vi "Link Channels.vi"(7 "gRPC ID in":T4, 8 "error in (no error)":errorcluster, 10 "Channels":T1[](array[typedef]), 11 "CIFCorePlugin in":refnum<class "CIFCorePlugin.lvclass">) -> (0 "error out":errorcluster, 3 "CIFCorePlugin out":refnum<class "CIFCorePlugin.lvclass">)   [LabVIEW 2021, in "Template Test Helpers.lvlib"]
uses:
  Template Test Helpers.lvlib
  <vilib>/CIF Foundation/CIF Core/CIFCore/Grpc/CIFCoreWrapper/CIFCoreWrapper.lvlib
  <vilib>/CIF Foundation/CIF Channels Core/ChannelCommon/ChannelCommon.lvlib
  <vilib>/CIF Foundation/CIF Channels Core/ChannelCommon/typedef/New FIFO Instance Configuration.ctl
  <vilib>/CIF Foundation/CIF Channels Core/CIFChannels/CIFChannels.lvclass
  <vilib>/CIF Foundation/CIF Core/CIFCore/Grpc/CIFCoreChannel_client/RPC Messages/cif_channelcore_ConnectSubscriber.ctl
  <vilib>/CIF Foundation/CIF Core/CIFCore/Grpc/CIFCoreChannel_client/CIFCoreChannel_client.lvlib
  <vilib>/CIF Foundation/CIF Core/CIFCore/Common/Typedef/FIFO Publisher.ctl
  <vilib>/CIF Foundation/CIF Core/CIFCore/Common/CIFCoreCommon.lvlib
  <vilib>/CIF Foundation/CIF Core/CIFCore/Class/CIFCorePlugin.lvclass
  <vilib>/gRPC/LabVIEW gRPC Library/Shared/grpcId.ctl
  <vilib>/gRPC/LabVIEW gRPC Library/grpc-lvsupport-release.lvlib
  <vilib>/CIF Foundation/CIF Core/CIFCore/Grpc/CIFCoreChannel_client/RPC Messages/cif_channelcore_PATTERN.ctl
  <vilib>/CIF Foundation/CIF Core/CIFCore/Grpc/CIFCoreChannel_client/RPC Messages/cif_channelcore_Direction.ctl
  <vilib>/CIF Foundation/CIF Core/CIFCore/Grpc/CIFCoreChannel_client/RPC Messages/cif_channelcore_Channel.ctl
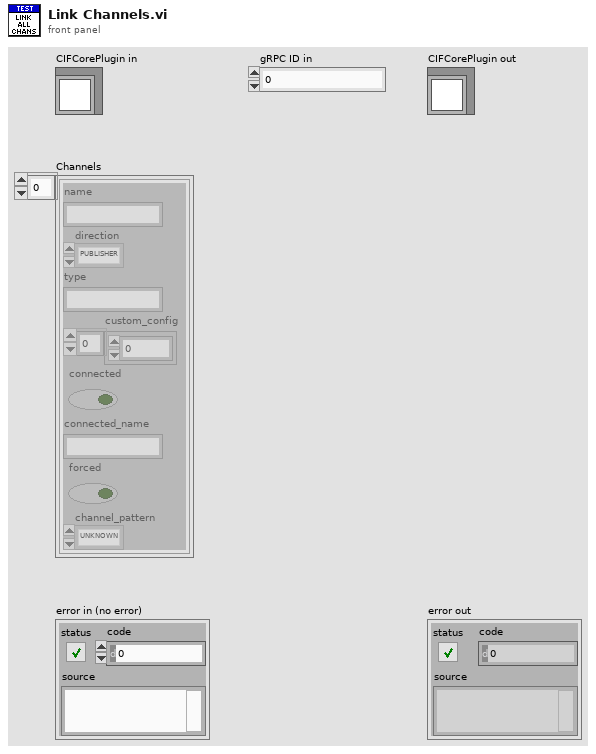
[diagram p1: front panel]
types:
  T1 = typedef "CIFCoreChannel_client.lvlib/cif_channelcore_Channel.ctl" = cluster{"name":string, "direction":T2, "type":string, "custom_config":u8[], "connected":bool, "connected_name":string, "forced":bool, "channel_pattern":T3}
  T2 = typedef "CIFCoreChannel_client.lvlib/cif_channelcore_Direction.ctl" = enum32{"PUBLISHER", "SUBSCRIBER"}
  T3 = typedef "CIFCoreChannel_client.lvlib/cif_channelcore_PATTERN.ctl" = enum32{"UNKNOWN", "TAG", "FIFO", "MULTIFIFO", "BACKPRESSUREFIFO"}
  T4 = typedef "grpc-lvsupport-release.lvlib/grpcId.ctl" = u64
  T5 = typedef "CIFCoreCommon.lvlib/FIFO Publisher.ctl" = cluster{"Publisher Name":string, "New FIFO Instance Config":T6}
  T6 = typedef "ChannelCommon.lvlib/New FIFO Instance Configuration.ctl" = cluster{"Backpressure":bool, "Bytes/Message Override":u32, "Messages/FIFO Override":u32, "Custom Data":u8[]}
  T7 = typedef "CIFCoreChannel_client.lvlib/cif_channelcore_ConnectSubscriber.ctl" = cluster{"subscriber_name":string, "publisher_name":string, "custom_connect":u8[]}
  T8 = typedef "CIFChannels.lvclass/Direction.ctl" = enum16{"Publisher", "Subscriber"}
  T9 = typedef "ChannelCommon.lvlib/FIFO Config.ctl" = cluster{"Max Bytes/Msg":u64, "Max Msg/FIFO":u64, "Flags":u64, "Custom Data":u8[]}
  T10 = typedef "ChannelCommon.lvlib/FIFO Flags.ctl" = cluster{"Backpressure":bool}
  T11 = typedef "ChannelCommon.lvlib/New FIFO Instance Response.ctl" = cluster{"Publisher":string, "Custom Data":u8[]}
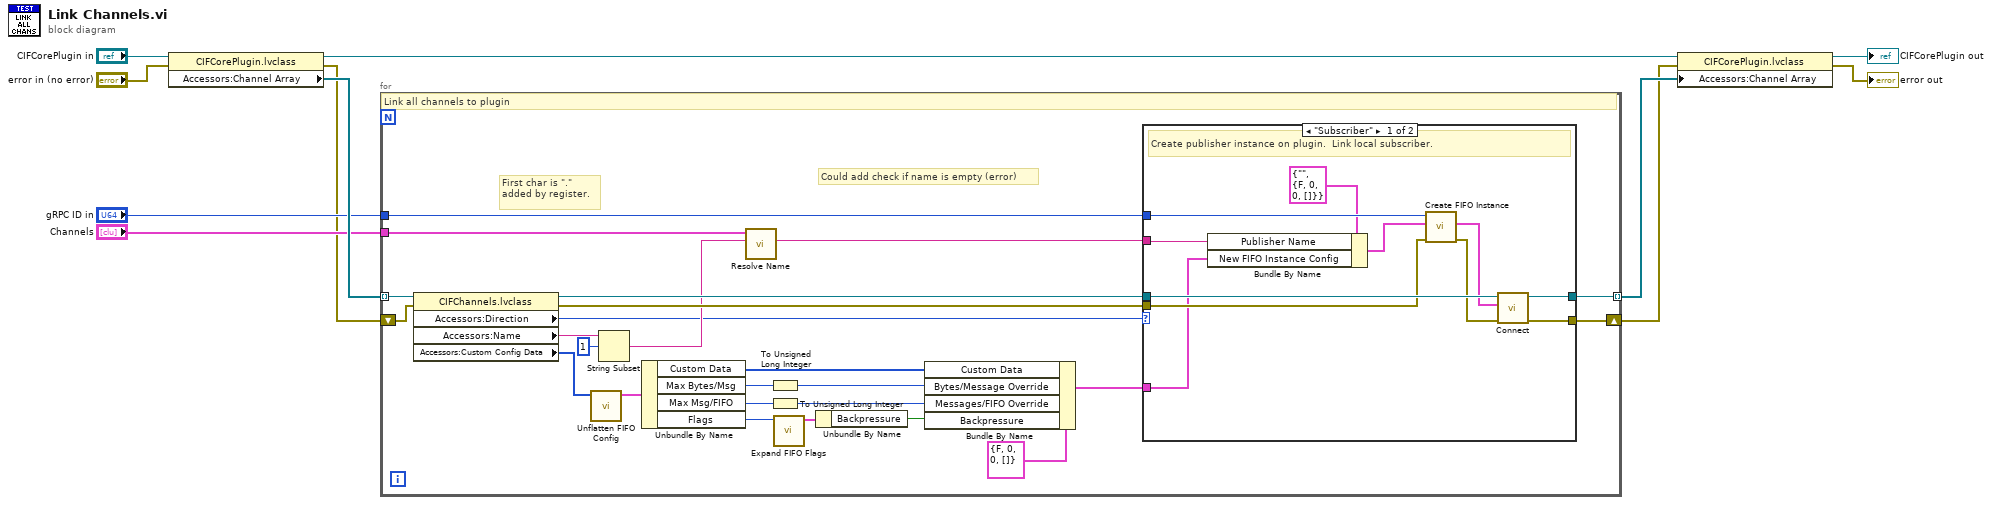
[diagram p0: block diagram]
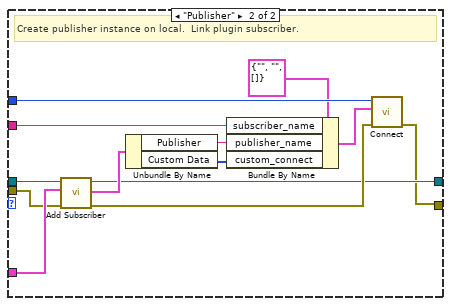
[diagram p2: hidden frame]
diagram:
  n1 = property class="CIFCorePlugin.lvclass"(reference="CIFCorePlugin in", error in="error in (no error)") -> (reference out=w5:refnum<class "CIFCorePlugin.lvclass">, error out=w6:errorcluster, "Accessors:Channel Array"=w10:refnum<class "CIFChannels.lvclass">[])
  n2 = for {
    tunnel: w10 -> [w35] mode=indexing
    tunnel: "Channels" -> [w32]
    tunnel: "gRPC ID in" -> [w31]
    tunnel: [w28] -> w4 mode=indexing
    shift-right: [w27] -> w2
    shift-left: w6 -> [w30]
    w14 = T6 {"Backpressure"=FALSE, "Bytes/Message Override"=0, "Messages/FIFO Override"=0, "Custom Data"=[]} ("New FIFO Instance Config")
    # "Could add check if name is empty (error)"
    # "First char is \".\" added by register."
    # "Link all channels to plugin"
    n3 = property class="CIFChannels.lvclass"(reference=w35, error in=w30) -> (reference out=w34:refnum<class "CIFChannels.lvclass">, error out=w29:errorcluster, "Accessors:Direction"=w15:T8, "Accessors:Name"=w13:string, "Accessors:Custom Config Data"=w33:u8[])
    n4 = call <vilib>:"Unflatten FIFO Config.vi"("Flattened Data in"=w33) -> ("FIFO Config out"=w26:T9)  [unwired: 9 in, 1 out]
    n5 = String Subset(string=w13, offset (0)=1) -> (substring=w16:string)  [unwired: 1 in]
    n6 = Unbundle By Name(w26) -> ("Custom Data"=w20:u8[], "Max Bytes/Msg"=w24:u64, "Max Msg/FIFO"=w23:u64, "Flags"=w25:u64)
    n7 = call <vilib>:"Resolve Name.vi"("Name in"=w16, "Channels"=w32) -> ("Name out"=w12:string)  [unwired: 8 in, 1 out]
    n8 = To Unsigned Long Integer(number=w24) -> (unsigned 32bit integer=w19:u32)
    n9 = To Unsigned Long Integer(number=w23) -> (unsigned 32bit integer=w18:u32)
    n10 = call <vilib>:"Expand FIFO Flags.vi"("FIFO Flags"=w25) -> ("Flags"=w22:T10)  [unwired: 10 in]
    n11 = Unbundle By Name(w22) -> ("Backpressure"=w21:bool)
    n12 = Bundle By Name(cluster=w14, "Custom Data"=w20, "Bytes/Message Override"=w19, "Messages/FIFO Override"=w18, "Backpressure"=w21) -> ()  [unwired: 1 out]
    n13 = case shown="\"Subscriber\"" w15 {
      tunnel: w34 -> [w46 w59]
      tunnel: w31 -> [w45 w58]
      tunnel: w29 -> [w44 w51]
      tunnel: [w43 w49] -> w28
      tunnel: [w42 w48] -> w27
      tunnel: w14 -> [w37 w57]
      tunnel: w12 -> [w38 w47]
      frame "Subscriber" {
        # "Create publisher instance on plugin.  Link local subscriber."
        n14 = Bundle By Name(cluster=T5 {"Publisher Name"="", "New FIFO Instance Config"={"Backpressure"=FALSE, "Bytes/Message Override"=0, "Messages/FIFO Override"=0, "Custom Data"=[]}} ("New Publisher"), "Publisher Name"=w38, "New FIFO Instance Config"=w37) -> (w36:T5)
        n15 = call <vilib>:"Create FIFO Instance.vi"("error in"=w44, "New Publisher"=w36, "gRPC ID"=w45) -> ("error out"=w41:errorcluster, "FIFO Instance"=w40:T11)  [unwired: 6 in, 1 out]
        n16 = call-dynamic <vilib>:"Connect.vi"("error in (no error)"=w41, "Connection"=w40, "CIFChannels in"=w46) -> ("error out"=w42:errorcluster, "CIFChannels out"=w43:refnum<class "CIFChannels.lvclass">)  [unwired: 7 in]
      }
      frame "Publisher" {
        # "Create publisher instance on local.  Link plugin subscriber."
        n17 = call-dynamic "Add Subscriber.vi"("error in (no error)"=w51, "New FIFO Instance Config"=w57, "CIFChannels in"=w59) -> ("error out"=w50:errorcluster, "New FIFO Instance"=w55:T11, "CIFChannels out"=w49:refnum<class "CIFChannels.lvclass">)  [unwired: 6 in]
        n18 = Unbundle By Name(w55) -> ("Publisher"=w54:string, "Custom Data"=w53:u8[])
        n19 = Bundle By Name(cluster=T7 {"subscriber_name"="", "publisher_name"="", "custom_connect"=[]} ("Connection"), "subscriber_name"=w47, "publisher_name"=w54, "custom_connect"=w53) -> (w52:T7)
        n20 = call <vilib>:"Connect.vi"("error in"=w50, "Connection"=w52, "gRPC ID"=w58) -> ("error out"=w48:errorcluster)  [unwired: 7 in, 1 out]
      }
    }
  }
  n21 = property class="CIFCorePlugin.lvclass"(reference=w5, error in=w2, "Accessors:Channel Array"=w4) -> (reference out=→"CIFCorePlugin out":refnum<class "CIFCorePlugin.lvclass">, error out=→"error out":errorcluster)
